vi "Status Heater (Read).vi"(6 "ISOBUS address":T3=-1 caption="ISOBUS address (-1)", 8 "error in":errorcluster, 11 "Mercury Reference In":T4) -> (0 "error out":errorcluster, 2 "State":T1, 3 "Mercury Reference Out":T4, 4 "Valid?":T2)   [LabVIEW 2018]
doc: "Read the output state of an output."
uses:
  Controls/Mercury Reference.ctl
  Controls/Comms Transport Layer.ctl
  Private/Controls/Query Dynamic Reference.ctl
  Controls/ISOBus Address.ctl
  Controls/Is Valid LED.ctl
  Controls/Unit String.ctl
  Private/Controls/Command Verbs.ctl
  Mercury iXX.lvlib
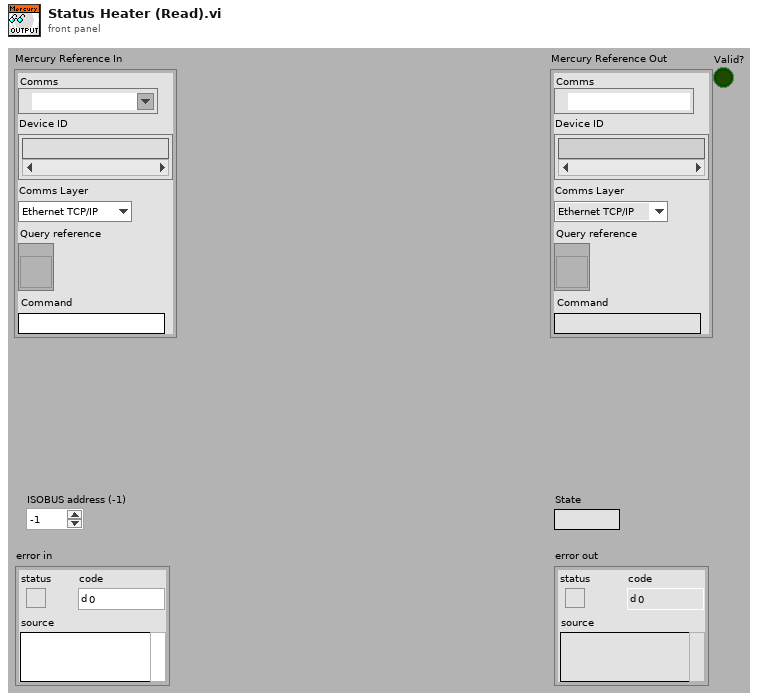
[diagram p1: front panel]
types:
  T1 = typedef "Mercury iXX.lvlib/Unit String.ctl" = string
  T2 = typedef "Mercury iXX.lvlib/Is Valid LED.ctl" = bool
  T3 = typedef "Mercury iXX.lvlib/ISOBus Address.ctl" = i32
  T4 = typedef "Mercury iXX.lvlib/Mercury Reference.ctl" = cluster{"Comms":refnum<visa-resource-name>, "Device ID":string[], "Comms Layer":T5, "Command":string, "Query reference":T6}
  T5 = typedef "Mercury iXX.lvlib/Comms Transport Layer.ctl" = enum16{"Ethernet TCP/IP", "USB", "ISOBus - RS-232", "GPIB"}
  T6 = typedef "Mercury iXX.lvlib/Query Dynamic Reference.ctl" = refnum<vi>
  T7 = typedef "Mercury iXX.lvlib/Command Verbs.ctl" = string
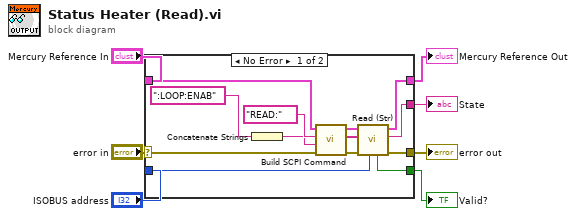
[diagram p0: block diagram]
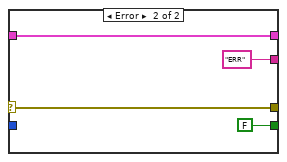
[diagram p2: hidden frame]
diagram:
  n1 = case shown="No Error" "error in" {
    selector: "error in" -> [w14 w23]
    tunnel: "Mercury Reference In" -> [w15 w24]
    tunnel: [w20 w23] -> w2
    tunnel: [w19 w24] -> w4
    tunnel: "ISOBUS address" -> [w18 _]
    tunnel: [w17 T2 FALSE ("Valid?")] -> w3
    tunnel: [w16 T1 "ERR" ("Unit")] -> w1
    frame No Error {
      n2 = Concatenate Strings(":LOOP:ENAB" ("Command")) -> (w8:string)
      n3 = call "Build SCPI Command.vi"("error in"=w14, "Noun(s)"=w8, "Verb"=T7 "READ:", "Mercury Reference In"=w15) -> ("error out"=w10:errorcluster, "SCPI Message(s)"=w9:string[], "Mercury Reference Out"=w13:T4)  [unwired: 5 out]
      n4 = call "Read (Str).vi"("ISOBUS address"=w18, "error in"=w10, "SCPI Message(s)"=w9, "Mercury Reference In"=w13) -> ("error out"=w20:errorcluster, "Response"=w16:string, "Mercury Reference Out"=w19:T4, "Valid?"=w17:T2)  [unwired: 4 out]
    }
    frame Error {
    }
  }
  "Mercury Reference Out" <- w4
  "Valid?" <- w3
  "error out" <- w2
  "State" <- w1
